vi "PID r-y windup.vi"(8 "Saturation":dbl[](array[numeric])=[-1.0, 1.0], 9 "Reverse Motor?":bool, 10 "PID Gains":cluster{"Kp":dbl, "Kd":dbl, "Ki":dbl}, 11 "Reference -\nEncoder position":dbl) -> (0 "Duty cycle":dbl, 1 "Windup (Ki Disable?)":bool, 2 "DIR":bool, 3 "Duty Cycle (Abs)":dbl)   [LabVIEW 2018]
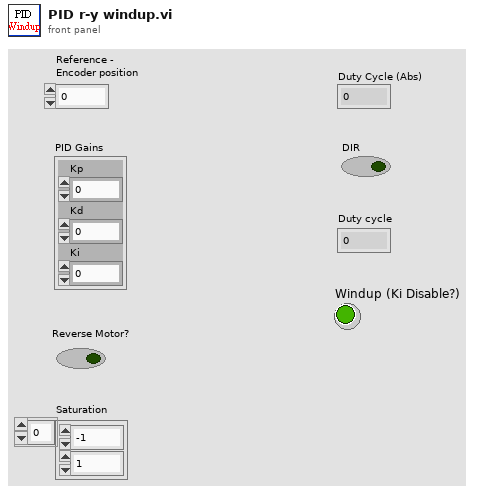
[diagram p1: front panel]
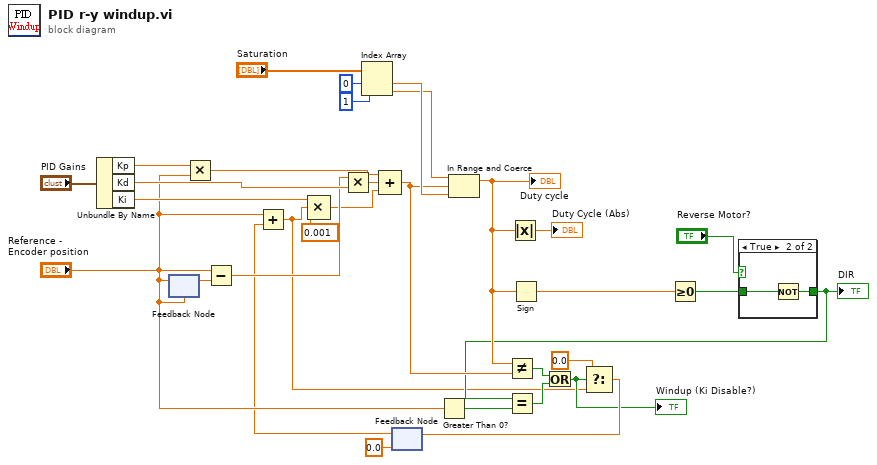
[diagram p0: block diagram]
diagram:
  n1 = Unbundle By Name("PID Gains") -> ("Kp"=w29:dbl, "Kd"=w32:dbl, "Ki"=w9:dbl)
  n2 = feedback #1("Reference -\nEncoder position") -> (w22:dbl)
  n3 = feedback-in #1("Reference -\nEncoder position") -> ()
  n4 = Multiply(x=w29, y="Reference -\nEncoder position") -> (x*y=w30:dbl)
  n5 = Subtract(x="Reference -\nEncoder position", y=w22) -> (x-y=w31:dbl)
  n6 = Multiply(x=w31, y=w32) -> (x*y=w13:dbl)
  n7 = Index Array(array="Saturation", index #1=0 ("index"), index #2=1 ("index")) -> (element #1=w24:dbl, element #2=w23:dbl)
  n8 = feedback #2(0.0 ("Ki")) -> (w3:dbl)
  n9 = Add(x="Reference -\nEncoder position", y=w3) -> (x+y=w1:dbl)
  n10 = Compound Arithmetic op=MULTIPLY(w9, w1, 0.001 ("value")) -> (w2:dbl)
  n11 = Compound Arithmetic op=ADD(w30, w13, w2) -> (w18:dbl)
  n12 = Greater Than 0?(x="Reference -\nEncoder position") -> (x > 0?=w6:bool)
  n13 = In Range and Coerce(upper limit=w23, x=w18, lower limit=w24) -> (coerced(x)=w19:dbl)  [unwired: 1 out]
  "Duty cycle" <- w19
  n14 = Not Equal?(x=w19, y=w18) -> (x != y?=w12:bool)
  n15 = Absolute Value(x=w19) -> (abs(x)=→"Duty Cycle (Abs)":dbl)
  n16 = Sign(1:w19) -> (0:w8:dbl)
  n17 = Greater Or Equal To 0?(x=w8) -> (x >= 0?=w7:bool)
  n18 = case shown="True" "Reverse Motor?" {
    tunnel: w7 -> [w33 w35]
    tunnel: [w33 w34] -> w5
    frame False {
    }
    frame True {
      n19 = Not(x=w35) -> (.not. x?=w34:bool)
    }
  }
  "DIR" <- w5
  n20 = Equal?(x=w5, y=w6) -> (x = y?=w11:bool)
  n21 = Or(x=w12, y=w11) -> (x .or. y?=w10:bool)
  "Windup (Ki Disable?)" <- w10
  n22 = Select(t=0.0, s=w10, f=w1) -> (s? t:f=w16:dbl)
  n23 = feedback-in #2(w16) -> ()
